vi "Wire Encode Varint I64.vi"(10 "I64":i64, 11 "Buffer in":u8[](array[numeric]) format="%.0x") -> (3 "Buffer":u8[](array[numeric]) format="%02x")   [LabVIEW 2020, in "LV-Proto.lvlib"]
uses:
  LV-Proto.lvlib
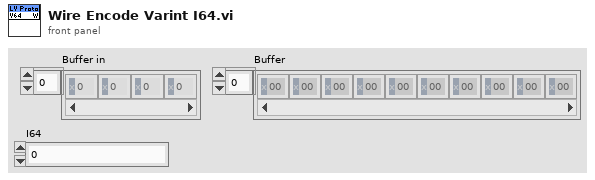
[diagram p1: front panel]
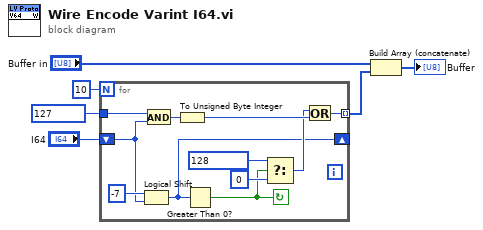
[diagram p0: block diagram]
diagram:
  n1 = for {
    N: 10 -> [_]
    shift-right: [w8] -> _
    shift-left: "I64" -> [w9]
    tunnel: i64 127 -> [w17]
    tunnel: [w7] -> w1 mode=indexing
    stop <- w11 continue-if-true
    n2 = Logical Shift(y=i16 -7, x=w9) -> (x << y=w8:i64)
    n3 = And(x=w17, y=w9) -> (x .and. y?=w15:i64)
    n4 = To Unsigned Byte Integer(number=w15) -> (unsigned 8bit integer=w14:u8)
    n5 = Greater Than 0?(x=w8) -> (x > 0?=w11:bool)
    n6 = Select(t=u8 128, s=w11, f=u8 0) -> (s? t:f=w10:u8)
    n7 = Or(x=w10, y=w14) -> (x .or. y?=w7:u8)
  }
  n8 = Build Array (concatenate)("Buffer in", w1) -> (→"Buffer":u8[])
